vi "SubpanelSimDataTemplate.vi"() -> ()   [LabVIEW 2016]
uses:
  Utilities/DataShare/DataShare.lvclass
panel:
  in  "Clear":bool
  in  "Filter":string
  in  "DataList":i32(listbox)
  out "Data":cluster{"X":dbl, "Y":dbl}[](graph)
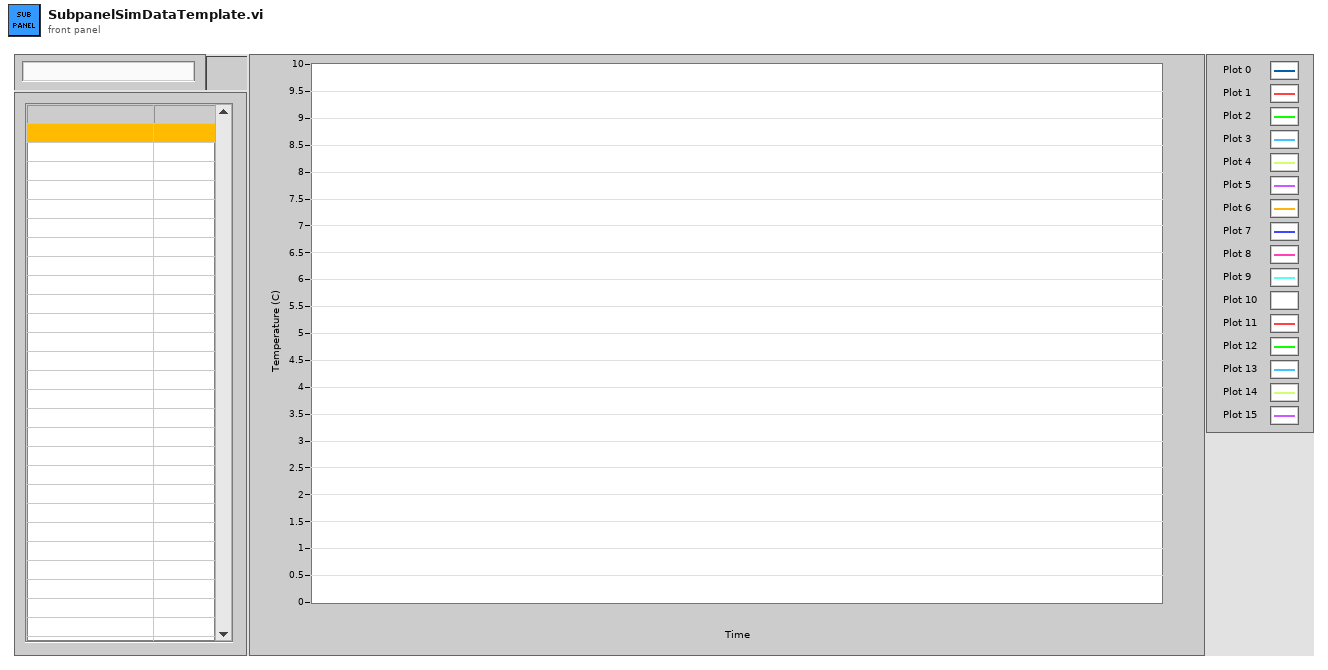
[diagram p1: front panel]
types:
  T1 = cluster{"Error":errorcluster, "SubpanelName":string, "DataShare":refnum<class "DataShare.lvclass">}
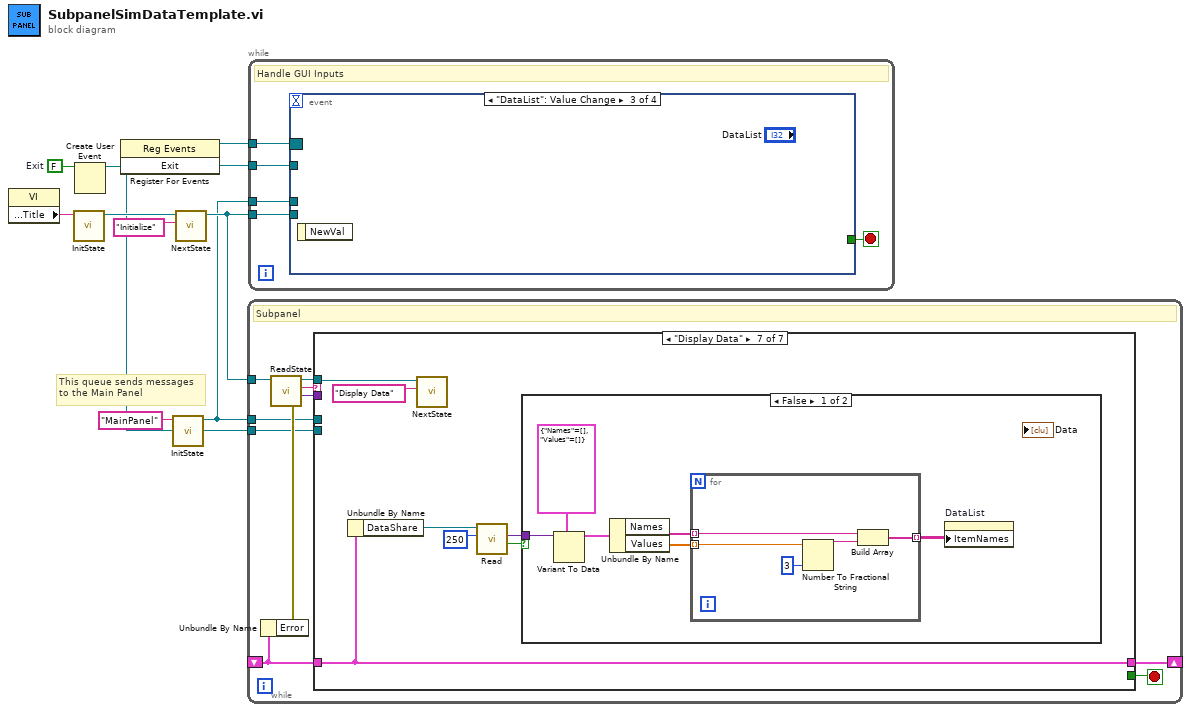
[diagram p0: block diagram]
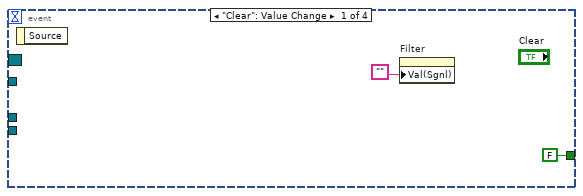
[diagram p2: hidden frame]
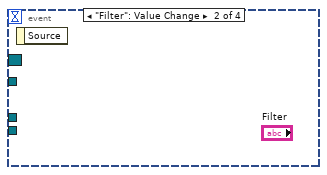
[diagram p3: hidden frame]
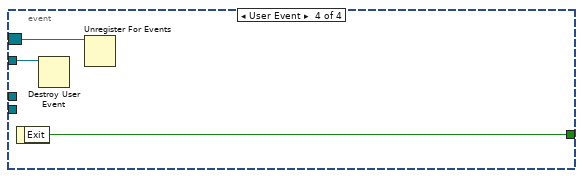
[diagram p4: hidden frame]
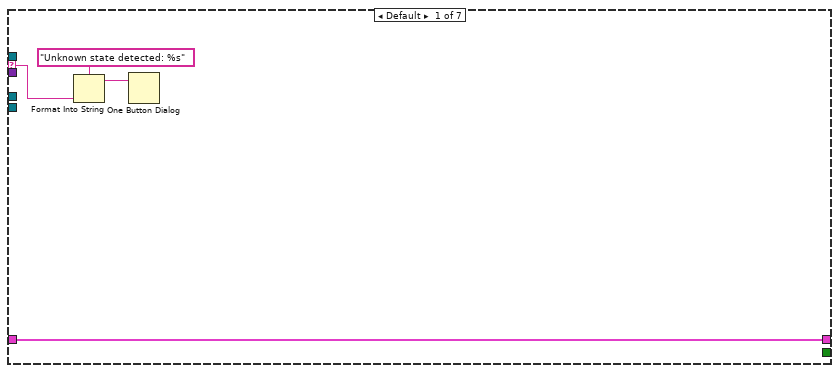
[diagram p5: hidden frame]
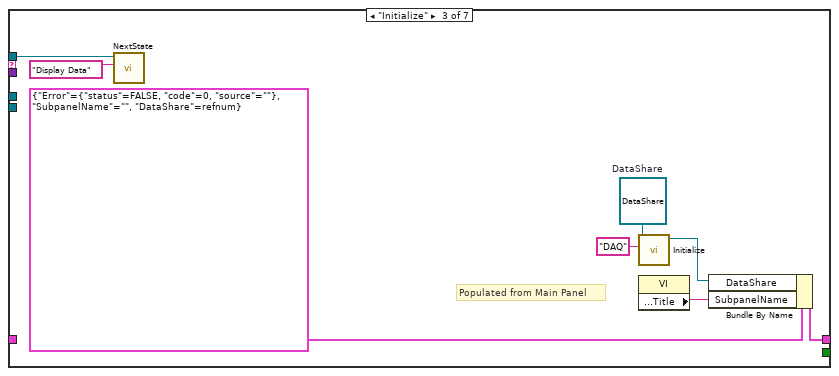
[diagram p7: hidden frame]
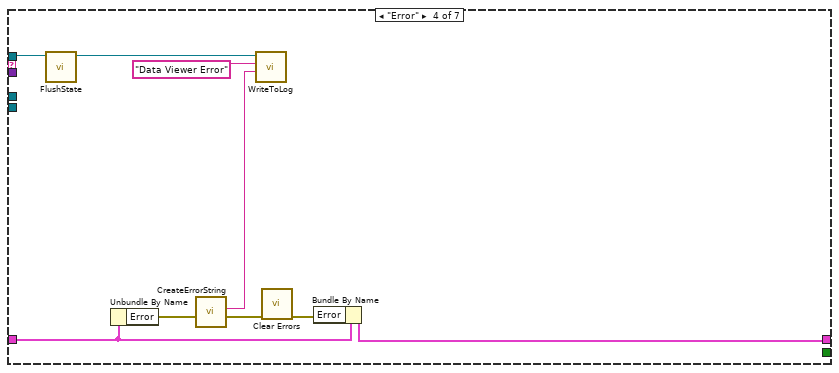
[diagram p8: hidden frame]
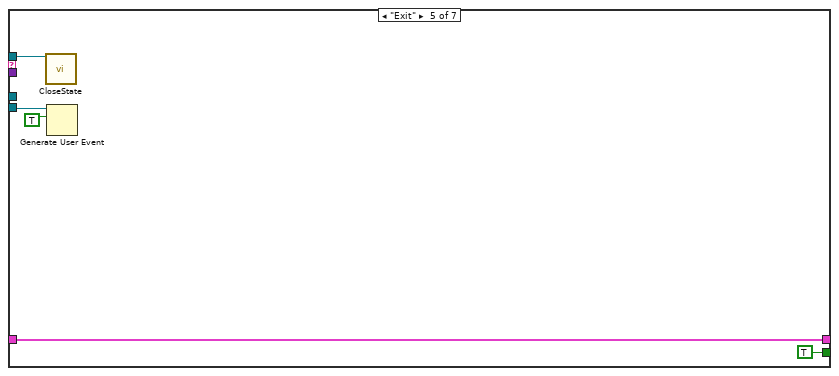
[diagram p9: hidden frame]
diagram:
  w3 = FALSE  # Exit
  # "This queue sends messages\nto the Main Panel"
  n1 = property class="VI"() -> ("Front Panel.Title"=w4:string)  [unwired: 2 in, 2 out]
  n2 = call "InitState.vi"("Name"=w4) -> ("Queue Out"=w9:refnum<queue>)  [unwired: 8 in, 1 out]
  n3 = Create User Event(user event datatype=w3) -> (user event=w1:refnum<user-event>)  [unwired: 1 in, 1 out]
  n4 = register-events(w1) -> (reference out=w2:refnum<event-registration>)  [unwired: 2 in, 1 out]
  n5 = call "InitState.vi"("Name"="MainPanel" ("name (unnamed)")) -> ("Queue Out"=w5:refnum<queue>)  [unwired: 8 in, 1 out]
  n6 = call "NextState.vi"("State"="Initialize" ("element"), "Queue In"=w9) -> ("Queue Out"=w7:refnum<queue>)  [unwired: 8 in, 1 out]
  n7 = while {
    tunnel: w7 -> [w17]
    shift-right: [w19] -> _
    shift-left: _ -> [w13]
    tunnel: w5 -> [w11]
    tunnel: w1 -> [w10]
    stop <- w18 stop-if-true
    # "Subpanel"
    n8 = Unbundle By Name(w13) -> ("Error"=w12:errorcluster)
    n9 = call "ReadState.vi"("Error In"=w12, "Queue In"=w17) -> ("Data"=w14:variant, "State"=w15:string, "Queue Out"=w16:refnum<queue>)  [unwired: 6 in, 1 out]
    n10 = case shown="\"Display Data\"" w15 {
      tunnel: w14 -> [_ _ _ _ _ _ _]
      selector: w15 -> [w22 _ _ _ _ _ _]
      tunnel: [w20 w24 w31 w41 w45 w47 w52] -> w19
      tunnel: [_ _ _ _ TRUE _ _] -> w18
      tunnel: w13 -> [w20 w24 _ w40 w45 w47 w52]
      tunnel: w16 -> [_ _ w26 w39 w44 _ w54]
      tunnel: w11 -> [_ _ _ _ _ _ _]
      tunnel: w10 -> [_ _ _ _ w43 _ _]
      frame Default {
        n11 = Format Into String(format string="Unknown state detected: %s", w22) -> (resulting string=w21:string)  [unwired: 2 in, 1 out]
        n12 = One Button Dialog(message=w21) -> ()  [unwired: 1 in, 1 out]
      }
      frame "--- System ---" {
      }
      frame "Initialize" {
        w25 = refnum<class "DataShare.lvclass"> refnum  # DataShare
        # "Populated from Main Panel"
        n13 = call "NextState.vi"("State"="Display Data" ("element"), "Queue In"=w26) -> ()  [unwired: 8 in, 2 out]
        n14 = call "Initialize.vi"("Name"="DAQ", "DataShare in"=w25) -> ("DataShare out"=w28:refnum<class "DataShare.lvclass">)  [unwired: 8 in, 1 out]
        n15 = property class="VI"() -> ("Front Panel.Title"=w30:string)  [unwired: 2 in, 2 out]
        n16 = Bundle By Name(cluster=T1 {"Error"={"status"=FALSE, "code"=0, "source"=""}, "SubpanelName"="", "DataShare"=refnum}, "DataShare"=w28, "SubpanelName"=w30) -> (w31:T1)
      }
      frame "Error" {
        n17 = call "FlushState.vi"("Queue In"=w39) -> ("Queue Out"=w38:refnum<queue>)  [unwired: 9 in, 1 out]
        n18 = Unbundle By Name(w40) -> ("Error"=w35:errorcluster)
        n19 = call "CreateErrorString.vi"("Error In"=w35) -> ("Error Out"=w34:errorcluster, "Error String"=w33:string)  [unwired: 9 in]
        n20 = call "WriteToLog.vi"("Data"=w33, "Source"="Data Viewer Error", "Queue In"=w38) -> ()  [unwired: 7 in, 2 out]
        n21 = call <vilib>:"Clear Errors.vi"("error in (no error)"=w34) -> ("error out"=w36:errorcluster)  [unwired: 5 in, 1 out]
        n22 = Bundle By Name(cluster=w40, "Error"=w36) -> (w41:T1)
      }
      frame "Exit" {
        n23 = call "CloseState.vi"("Queue In"=w44) -> ()  [unwired: 10 in, 1 out]
        n24 = Generate User Event(user event=w43, event data cluster=TRUE ("event data")) -> ()  [unwired: 2 in, 2 out]
      }
      frame "--- Process Telemetry ---" {
      }
      frame "Display Data" {
        n25 = Unbundle By Name(w52) -> ("DataShare"=w51:refnum<class "DataShare.lvclass">)
        n26 = call "NextState.vi"("State"="Display Data" ("element"), "Queue In"=w54) -> ()  [unwired: 8 in, 2 out]
        n27 = call "Read.vi"("Timeout"=250, "DataShare in"=w51) -> ("Timed Out?"=w49:bool, "Data"=w48:variant)  [unwired: 6 in, 2 out]
        n28 = case shown="False" w49 {
          tunnel: w48 -> [w60 _]
          frame False {
            n29 = Variant To Data(type=cluster{"Names":string[], "Values":dbl[]} {"Names"=[], "Values"=[]}, Variant=w60) -> (data=w58:cluster{"Names":string[], "Values":dbl[]})  [unwired: 1 in, 1 out]
            n30 = Unbundle By Name(w58) -> ("Names"=w57:string[], "Values"=w56:dbl[])
            n31 = for {
              tunnel: w57 -> [w63] mode=indexing
              tunnel: w56 -> [w62] mode=indexing
              tunnel: [w61] -> w55 mode=indexing
              n32 = Number To Fractional String(number=w62, precision (6)=i16 3) -> (F-format string=w64:string)  [unwired: 2 in]
              n33 = Build Array(w63, w64) -> (w61:string[])
            }
            n34 = property on="DataList" class="MCListbox (strict)"("ItemNames"=w55) -> ()  [unwired: 2 in, 2 out]
          }
          frame True {
          }
        }
      }
    }
  }
  n35 = while {
    tunnel: w7 -> [w70]
    tunnel: w5 -> [w68]
    tunnel: w2 -> [w67]
    tunnel: w1 -> [w66]
    stop <- w69 stop-if-true
    # "Handle GUI Inputs"
    n36 = event shown="[2] \"DataList\": Value Change" {
      selector: w67 -> [_ _ _ w74]
      dyn-events: _ -> [_ _ _ _]
      timeout: _ -> [_ _ _ _]
      tunnel: w70 -> [_ _ _ _]
      tunnel: [FALSE _ _ w73] -> w69
      tunnel: w68 -> [_ _ _ _]
      tunnel: w66 -> [_ _ _ w75]
      event "Clear": Value Change {
        n37 = event-data() -> ()  [unwired: 1 in, 1 out]
        n38 = property on="Filter" class="Str"("Val(Sgnl)"="") -> ()  [unwired: 2 in, 2 out]
      }
      event "Filter": Value Change {
        n39 = event-data() -> ()  [unwired: 1 in, 1 out]
      }
      event "DataList": Value Change {
        n40 = event-data() -> ()  [unwired: 1 in, 1 out]
      }
      event User Event {
        n41 = event-data() -> ("Exit"=w73:bool)  [unwired: 1 in]
        n42 = Destroy User Event(user event=w75) -> ()  [unwired: 1 in, 1 out]
        n43 = Unregister For Events(event registration refnum=w74) -> ()  [unwired: 1 in, 1 out]
      }
    }
  }
